vi "Stepper ToGo.vi"(8 "error in":errorcluster, 11 "Arduino Resource":T1={"VISA resource"="", "Board Type"=enum."Uno", "Connection Type"=enum."USB / Serial", "Bytes Per Packet (15)"=15}) -> (0 "error out":errorcluster, 1 "Steps remaining":u16, 2 "Steps Remaining?":bool, 3 "Arduino Resource Out":T1={"VISA resource"="", "Board Type"=enum."Uno", "Connection Type"=enum."USB / Serial", "Bytes Per Packet (15)"=15})   [LabVIEW 2015, in "LabVIEW Interface for Arduino.lvlib"]
doc: "Check to see if the Arduino is still processing a previous step command. Wait until Steps Remaining? is false to ensure step commands aren't overwritten."
uses:
  <vilib>/LabVIEW Interface for Arduino/LabVIEW Interface for Arduino.lvlib
  <vilib>/LabVIEW Interface for Arduino/Type Defs/Arduino Resource.ctl
  <vilib>/LabVIEW Interface for Arduino/Type Defs/Board Type.ctl
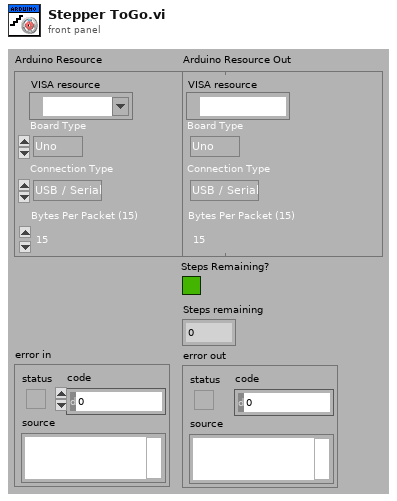
[diagram p1: front panel]
types:
  T1 = typedef "LabVIEW Interface for Arduino.lvlib/Arduino Resource.ctl" = cluster{"VISA resource":refnum<visa-resource-name>, "Board Type":T2, "Connection Type":enum8{"USB / Serial"}, "Bytes Per Packet (15)":u8}
  T2 = typedef "LabVIEW Interface for Arduino.lvlib/Board Type.ctl" = enum16{"Uno", "Dimuelanove w/Atmega 328", "Mega 2560"}
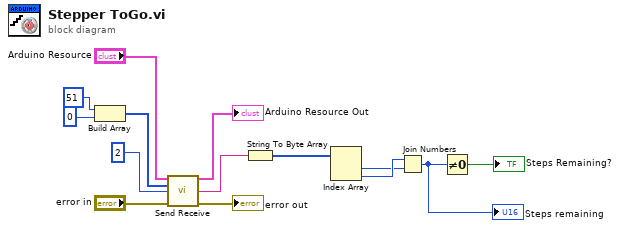
[diagram p0: block diagram]
diagram:
  n1 = Build Array(u8 51, u8 0 ("element")) -> (w8:u8[])
  n2 = call <vilib>:"Send Receive.vi"("Arduino Resource"="Arduino Resource", "Data"=w8, "Bytes To Read (0)"=u8 2, "error in"="error in") -> ("Arduino Resource"=→"Arduino Resource Out":T1, "Read Buffer"=w7:string, "error out"=→"error out":errorcluster)  [unwired: 9 in]
  n3 = String To Byte Array(string=w7) -> (unsigned byte array=w6:u8[])
  n4 = Index Array(array=w6) -> (element #1=w3:u8, element #2=w4:u8)  [unwired: 2 in]
  n5 = Join Numbers(hi=w4, lo=w3) -> ((hi.lo)=w1:u16)
  "Steps remaining" <- w1
  n6 = Not Equal To 0?(x=w1) -> (x != 0?=→"Steps Remaining?":bool)
